vi "DIAdem Process Script Request.vi"(5 "error in (no error)":errorcluster, 7 "DIAdem Queue":T1, 8 "DIAdem Reference":T3) -> (0 "error out":errorcluster, 2 "Script Result":string, 3 "DIAdem Reference":T3)   [LabVIEW 2011]
uses:
  <vilib>/ExportToExcel/DIAdem Reference.ctl
  DIAdem Daemon Queue.ctl
  DIAdem Daemon Script Type.ctl
  DIAdem Toolkit EXT/DIAdem.llb/DIAdem String Variable Set.vi
  <vilib>/ExportToExcel/DIAdem String Variable Get.vi
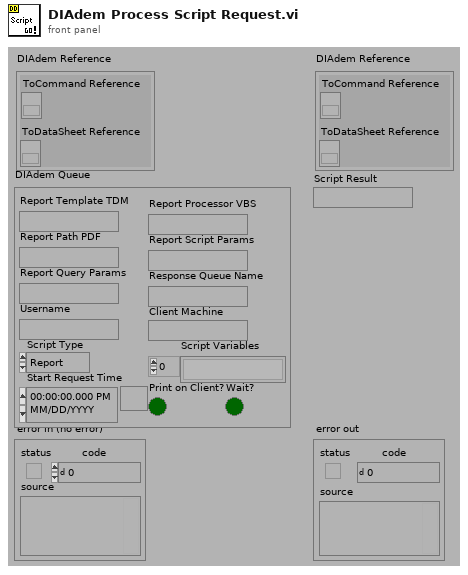
[diagram p1: front panel]
types:
  T1 = typedef "DIAdem Daemon Queue.ctl" = cluster{"Report Template TDM":path, "Report Processor VBS":path, "Report Path PDF":path, "Report Script Params":string, "Username":string, "Script Type":T2, "Report Query Params":string, "Client Machine":string, "Print on Client?":bool, "Response Queue Name":string, "Script Variables":string[], "Start Request Time":timestamp, "Wait?":bool}
  T2 = typedef "DIAdem Daemon Script Type.ctl" = enum16{"Report", "Query", "Script", "Datasheet", "Append", "Restart", "Stop"}
  T3 = typedef "DIAdem Reference.ctl" = cluster{"ToCommand Reference":refnum<k7>, "ToDataSheet Reference":refnum<k7>}
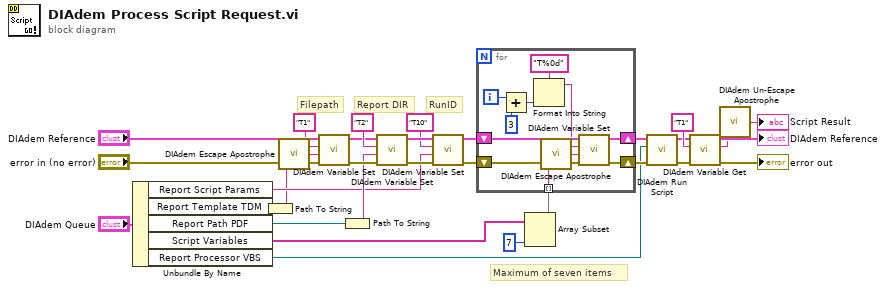
[diagram p0: block diagram]
diagram:
  # "Maximum of seven items"
  # "Report DIR"
  # "Filepath"
  # "RunID"
  n1 = Unbundle By Name("DIAdem Queue") -> ("Report Script Params"=w9:string, "Report Template TDM"=w30:path, "Report Path PDF"=w21:path, "Script Variables"=w17:string[], "Report Processor VBS"=w6:path)
  n2 = Path To String(path=w30) -> (string=w5:string)
  n3 = call "DIAdem Escape Apostrophe.vi"("String"=w5) -> ("Escaped String"=w4:string)
  n4 = call-poly "DIAdem Variable Set.vi"("error in (no error)"="error in (no error)", "Value"=w4, "Variable Name"="T1", "DIAdem Reference"="DIAdem Reference") -> ("error out"=w24:errorcluster, "DIAdem Reference"=w25:T3)  [unwired: 6 out]
  n5 = Path To String(path=w21) -> (string=w20:string)
  n6 = call-poly "DIAdem Variable Set.vi"("error in (no error)"=w24, "Value"=w20, "Variable Name"="T2", "DIAdem Reference"=w25) -> ("error out"=w13:errorcluster, "DIAdem Reference"=w14:T3)  [unwired: 6 out]
  n7 = call-poly "DIAdem Variable Set.vi"("error in (no error)"=w13, "Value"=w9, "Variable Name"="T10", "DIAdem Reference"=w14) -> ("error out"=w12:errorcluster, "DIAdem Reference"=w11:T3)  [unwired: 6 out]
  n8 = Array Subset(array=w17, length=7) -> (w1:string[])  [unwired: 1 in]
  n9 = for {
    shift-right: [w39] -> w18
    shift-left: w12 -> [w40]
    shift-right: [w42] -> w15
    shift-left: w11 -> [w41]
    tunnel: w1 -> [w32] mode=indexing
    i -> [w38]
    n10 = Add(x=w38, y=3) -> (x+y=w35:i32)
    n11 = Format Into String(format string="T%0d", w35) -> (resulting string=w34:string)  [unwired: 2 in, 1 out]
    n12 = call "DIAdem Escape Apostrophe.vi"("String"=w32) -> ("Escaped String"=w33:string)
    n13 = call-poly "DIAdem Variable Set.vi"("error in (no error)"=w40, "Value"=w33, "Variable Name"=w34, "DIAdem Reference"=w41) -> ("error out"=w39:errorcluster, "DIAdem Reference"=w42:T3)  [unwired: 6 out]
  }
  n14 = call "DIAdem Run Script.vi"("error in (no error)"=w18, "script file"=w6, "DIAdem Reference"=w15) -> ("error out"=w23:errorcluster, "DIAdem Reference"=w22:T3)  [unwired: 7 out]
  n15 = call-poly "DIAdem Variable Get.vi"("error in (no error)"=w23, "Variable Name"="T1", "DIAdem Reference"=w22) -> ("error out"=→"error out":errorcluster, "Value"=w3:string, "DIAdem Reference"=→"DIAdem Reference":T3)  [unwired: 6 out]
  n16 = call "DIAdem Un-Escape Apostrophe.vi"("Escaped String"=w3) -> ("String"=→"Script Result":string)
